vi "test.vi"() -> ()   [LabVIEW 2013]
panel:
  out "XY Graph":cluster{dbl[], dbl[]}[](graph)
  in  "Ts (ms)":dbl format="%#_13g"
  out "Time (s)":i32
  in  "stop":bool
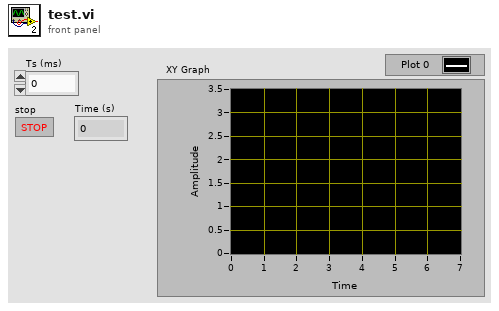
[diagram p1: front panel]
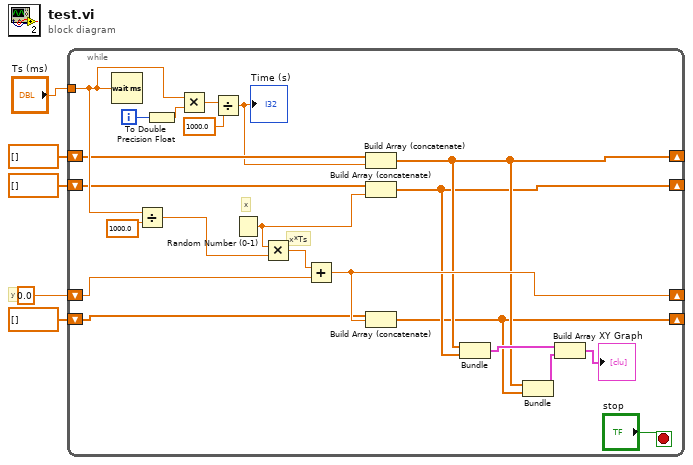
[diagram p0: block diagram]
diagram:
  # "y"
  n1 = while {
    shift-right: [w13] -> _
    shift-left: 0.0 -> [w18]
    tunnel: "Ts (ms)" -> [w22]
    shift-right: [w9] -> _
    shift-left: dbl[] [] -> [w17]
    shift-right: [w8] -> _
    shift-left: dbl[] [] -> [w15]
    shift-right: [w7] -> _
    shift-left: dbl[] [] -> [w12]
    i -> [w26]
    stop <- "stop" stop-if-true
    # "x*Ts"
    # "x"
    n2 = Wait (ms)(milliseconds to wait=w22) -> ()  [unwired: 1 out]
    n3 = Divide(x=w22, y=1000.0) -> (x/y=w20:dbl)
    n4 = To Double Precision Float(number=w26) -> (double precision float=w25:dbl)
    n5 = Multiply(x=w22, y=w25) -> (x*y=w24:dbl)
    n6 = Divide(x=w24, y=1000.0) -> (x/y=w16:dbl)
    "Time (s)" <- w16
    n7 = Random Number (0-1)() -> (number: 0 to 1=w14:dbl)
    n8 = Multiply(x=w14, y=w20) -> (x*y=w19:dbl)
    n9 = Add(x=w19, y=w18) -> (x+y=w13:dbl)
    n10 = Build Array (concatenate)(w17, w16) -> (w9:dbl[])
    n11 = Build Array (concatenate)(w15, w14) -> (w8:dbl[])
    n12 = Build Array (concatenate)(w12, w13) -> (w7:dbl[])
    n13 = Bundle(w9, w8) -> (w11:cluster{dbl[], dbl[]})  [unwired: 1 in]
    n14 = Bundle(w9, w7) -> (w10:cluster{dbl[], dbl[]})  [unwired: 1 in]
    n15 = Build Array(w11, w10) -> (→"XY Graph":cluster{dbl[], dbl[]}[])
  }
